vi "Ex2Cameras.vi"() -> ()   [LabVIEW 2010]
panel:
  in  "camera 2 name":string
  in  "camera 1 name":string
  in  "Store 2":bool
  in  "stop 2":bool
  in  "Store":bool
  in  "stop":bool
  in  "Intensifier Camera 2":bool
  in  "Intensifier Camera 1":bool
  in  "Exposure Camera 2":dbl=0.5 format="%.2f"
  in  "Exposure Camera 1":dbl=0.5 format="%.2f"
  out "error out":errorcluster
  in  "error in (no error)":errorcluster
  # "Ex2Cameras:\nThis example runs two cameras in focus mode.\nRemember to setup two cameras in the pvcam.ini\nfile."
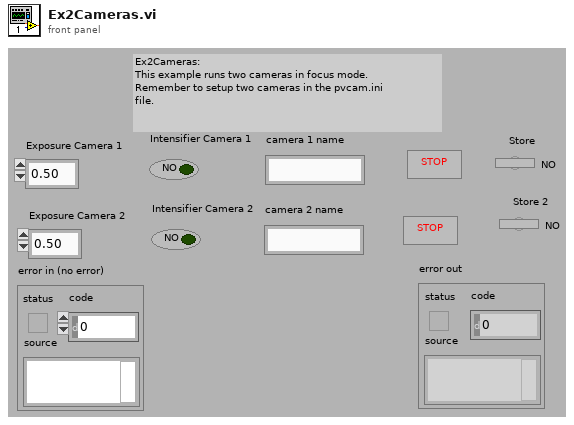
[diagram p1: front panel]
types:
  T1 = cluster{"Camera Handle":u32, "Pulser Handle":u32, "File Handle":u32, "Display Handle":u32, "Image Handle":u32}
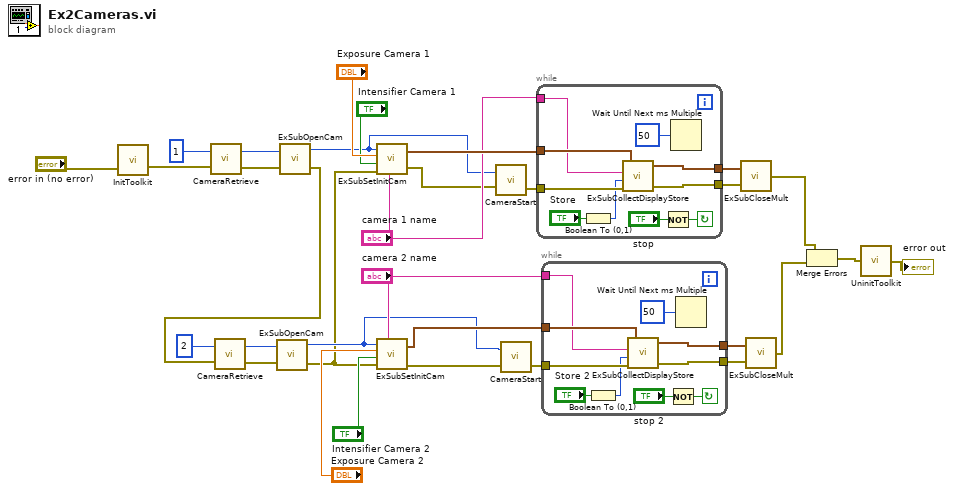
[diagram p0: block diagram]
diagram:
  n1 = call <userlib>:"InitToolkit.vi"("error in"="error in (no error)") -> ("error out"=w6:errorcluster)
  n2 = call <userlib>:"CameraRetrieve.vi"("error in"=w6, "Camera Index"=1) -> ("error out"=w8:errorcluster, "Device ID"=w7:u32)
  n3 = call "ExSubOpenCam.vi"("error in (no error)"=w8, "Camera Device ID"=w7) -> ("error out"=w2:errorcluster, "Camera Handle"=w18:u32)
  n4 = call <userlib>:"CameraRetrieve.vi"("error in"=w2, "Camera Index"=2) -> ("error out"=w3:errorcluster, "Device ID"=w4:u32)
  n5 = call "ExSubOpenCam.vi"("error in (no error)"=w3, "Camera Device ID"=w4) -> ("error out"=w9:errorcluster, "Camera Handle"=w17:u32)
  n6 = call "ExSubSetInitCam.vi"("Camera Handle"=w18, "Exposure"="Exposure Camera 1", "Intensifier"="Intensifier Camera 1", "error in (no error)"=w9, "Name"="camera 1 name") -> ("Handles Out"=w21:T1, "error out"=w12:errorcluster)
  n7 = call "ExSubSetInitCam.vi"("Camera Handle"=w17, "Exposure"="Exposure Camera 2", "Intensifier"="Intensifier Camera 2", "error in (no error)"=w9, "Name"="camera 2 name") -> ("Handles Out"=w22:T1, "error out"=w11:errorcluster)
  n8 = call <userlib>:"CameraStart.vi"("error in"=w12, "Camera Handle"=w18) -> ("error out"=w10:errorcluster)  [unwired: 1 out]
  n9 = call <userlib>:"CameraStart.vi"("error in"=w11, "Camera Handle"=w17) -> ("error out"=w23:errorcluster)  [unwired: 1 out]
  n10 = while {
    tunnel: w21 -> [w41]
    tunnel: w10 -> [w40]
    tunnel: "camera 1 name" -> [w33]
    tunnel: [w38] -> w26
    tunnel: [w39] -> w27
    stop <- w36 continue-if-true
    n11 = Boolean To (0,1)(Boolean="Store") -> (0, 1=w34:i16)
    n12 = call "ExSubCollectDisplayStore.vi"("error in (no error)"=w40, "Store flag"=w34, "Display Title"=w33, "Handle Cluster"=w41) -> ("error out"=w38:errorcluster, "Handle Cluster Out"=w39:T1)  [unwired: 1 out]
    n13 = Not(x="stop") -> (.not. x?=w36:bool)
    n14 = Wait Until Next ms Multiple(millisecond multiple=u32 50) -> ()  [unwired: 1 out]
  }
  n15 = while {
    tunnel: w22 -> [w51]
    tunnel: w23 -> [w50]
    tunnel: "camera 2 name" -> [w43]
    tunnel: [w48] -> w24
    tunnel: [w49] -> w25
    stop <- w46 continue-if-true
    n16 = Boolean To (0,1)(Boolean="Store 2") -> (0, 1=w44:i16)
    n17 = call "ExSubCollectDisplayStore.vi"("error in (no error)"=w50, "Store flag"=w44, "Display Title"=w43, "Handle Cluster"=w51) -> ("error out"=w48:errorcluster, "Handle Cluster Out"=w49:T1)  [unwired: 1 out]
    n18 = Not(x="stop 2") -> (.not. x?=w46:bool)
    n19 = Wait Until Next ms Multiple(millisecond multiple=u32 50) -> ()  [unwired: 1 out]
  }
  n20 = call "ExSubCloseMult.vi"("error in (no error)"=w26, "Handles In"=w27) -> ("error out"=w14:errorcluster)
  n21 = call "ExSubCloseMult.vi"("error in (no error)"=w24, "Handles In"=w25) -> ("error out"=w13:errorcluster)
  n22 = Merge Errors(w14, w13) -> (w16:errorcluster)
  n23 = call <userlib>:"UninitToolkit.vi"("error in"=w16) -> ("error out"=→"error out":errorcluster)
